vi "Drfit_check.vi"() -> ()   [LabVIEW 2019]
uses:
  <vilib>/eio/EIONode/EIONode.xnode
  <vilib>/rvi/eio/common/nirviEmuTemplateMethod_errors.vi
  <vilib>/rvi/DataTransferAndStorage/Container/XNode/niFpgaContainer.xnode
  <vilib>/rvi/FIFO/Fifo_Resource/nirvififoEmulationRead.vi
  <vilib>/eio/EIOPropertyNode/EIOPropertyNode.xnode
  <vilib>/rvi/eio/common/nirviEmuTemplatePropertyGet_errors.vi
  <vilib>/rvi/eio/common/nirviEmuTemplatePropertyGet_noerrors.vi
  <vilib>/rvi/eio/common/nirviEmuTemplatePropertySet_errors.vi
  <vilib>/rvi/eio/common/nirviEmuTemplatePropertySet_noerrors.vi
  <vilib>/rvi/FIFO/Fifo_Resource/nirvififoEmulationWrite.vi
  <vilib>/rvi/interface/RandomDataEmulation/nirviRandomDataFpgaReadWriteTemplate.vi
panel:
  in  "MobX(px/V)":sgl
  in  "1/Xcali":sgl
  in  "Xmean":sgl
  in  "Frequency":u32=100000
  in  "Triangle wave":T1={"signal offset_X"=5.0, "Scale X"=0.0, "signal offset_Y"=5.0, "Scale Y"=0.0, "Phase Shift"=30}
  in  "1/Ycali":sgl
  in  "Xoffset":sgl
  in  "Yoffset":sgl
  in  "sum_offset":sgl
  in  "Normalize signal":bool=TRUE
  in  "FB Time":u8=5 caption="Feedback loop time"
  out "Saveloop":u32
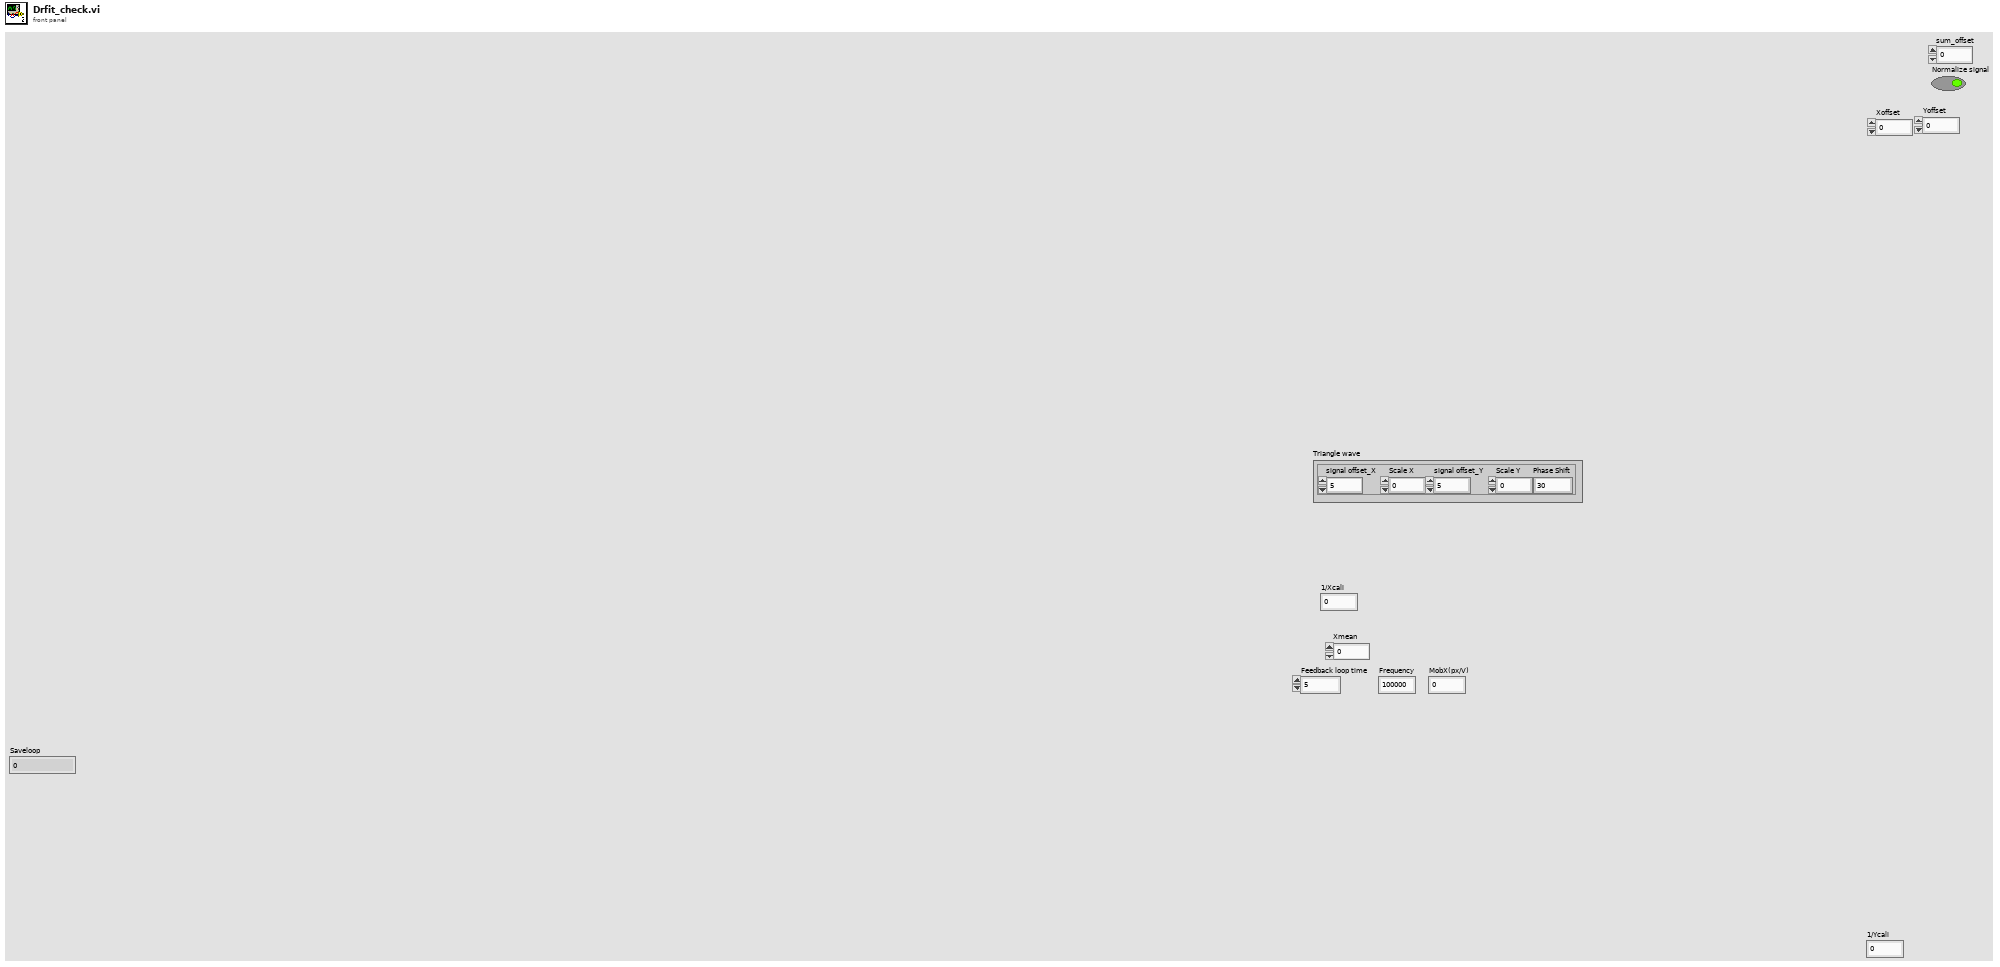
[diagram p1: front panel]
types:
  T1 = cluster{"signal offset_X":sgl, "Scale X":sgl, "signal offset_Y":sgl, "Scale Y":sgl, "Phase Shift":u32}
  T2 = enum8{"+/- 10 V", "+/- 5 V", "+/- 2 V", "+/- 1 V"}
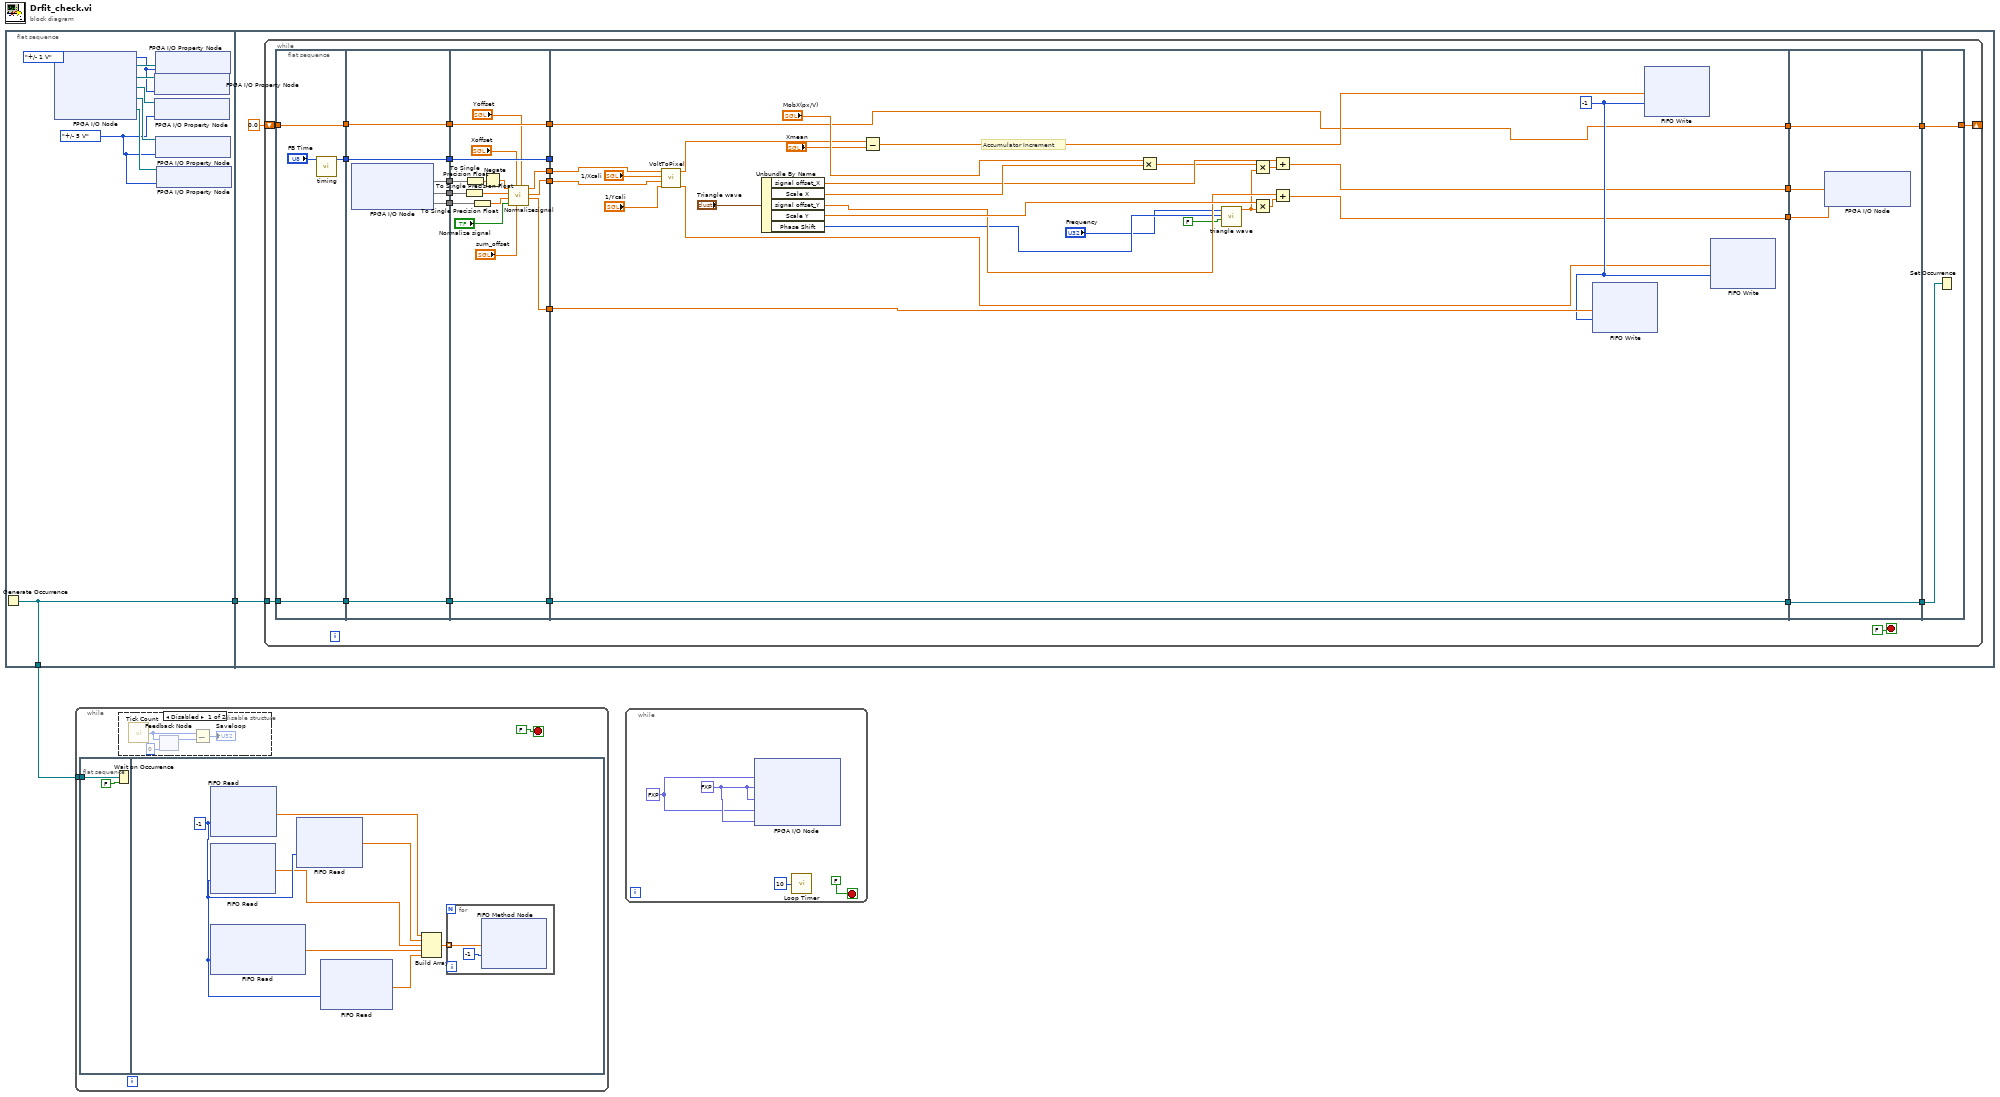
[diagram p0: block diagram]
diagram:
  n1 = flat-sequence {
    tunnel: [w3] -> w2
    tunnel: [w3] -> w1
    tunnel: w2 -> [w12]
    frame #0 {
      w4 = T2."+/- 5 V" ("Voltage Range")
      w7 = T2."+/- 1 V" ("Voltage Range")
      n2 = Generate Occurrence() -> (w3:refnum<k4>)
      n3 = xnode "FPGA I/O Node"() -> ("FPGA I/O Out"=w10:refnum<k21>, "FPGA I/O Out"=w8:refnum<k21>, "FPGA I/O Out"=w9:refnum<k21>, "FPGA I/O Out"=w5:refnum<k21>, "FPGA I/O Out"=w6:refnum<k21>)  [unwired: 5 in, 5 out]
      n4 = xnode "FPGA I/O Property Node"("FPGA I/O In"=w8, "Voltage Range"=w7) -> ()  [unwired: 1 out]
      n5 = xnode "FPGA I/O Property Node"("FPGA I/O In"=w9, "Voltage Range"=w4) -> ()  [unwired: 1 out]
      n6 = xnode "FPGA I/O Property Node"("FPGA I/O In"=w10, "Voltage Range"=w7) -> ()  [unwired: 1 out]
      n7 = xnode "FPGA I/O Property Node"("FPGA I/O In"=w5, "Voltage Range"=w4) -> ()  [unwired: 1 out]
      n8 = xnode "FPGA I/O Property Node"("FPGA I/O In"=w6, "Voltage Range"=w4) -> ()  [unwired: 1 out]
    }
    frame #1 {
      n9 = while {
        tunnel: w12 -> [w25]
        shift-right: [w17] -> _
        shift-left: sgl 0.0 -> [w15]
        stop <- FALSE ("stop") stop-if-true
        n10 = flat-sequence {
          tunnel: [w40] -> w26
          tunnel: w25 -> [w39]
          tunnel: [w39] -> w24
          tunnel: [w38] -> w16
          tunnel: w15 -> [w38]
          tunnel: [w47] -> w36
          tunnel: [w46] -> w34
          tunnel: [w45] -> w32
          tunnel: [w44] -> w27
          tunnel: w26 -> [w44]
          tunnel: w24 -> [w43]
          tunnel: [w43] -> w23
          tunnel: w16 -> [w42]
          tunnel: [w42] -> w13
          tunnel: w36 -> [w54]
          tunnel: [w63] -> w35
          tunnel: w34 -> [w53]
          tunnel: [w62] -> w33
          tunnel: w32 -> [w51]
          tunnel: [w61] -> w31
          tunnel: [w64] -> w28
          tunnel: w27 -> [w64]
          tunnel: w23 -> [w60]
          tunnel: [w60] -> w22
          tunnel: [w58] -> w14
          tunnel: w13 -> [w58]
          tunnel: w35 -> [w90]
          tunnel: w33 -> [w73]
          tunnel: w31 -> [w89]
          tunnel: [w74] -> w30
          tunnel: [w71] -> w29
          tunnel: w28 -> [_]
          tunnel: w22 -> [w87]
          tunnel: [w87] -> w20
          tunnel: [w82] -> w19
          tunnel: w14 -> [w82]
          tunnel: w29 -> [w94]
          tunnel: w30 -> [w95]
          tunnel: [w93] -> w21
          tunnel: w20 -> [w93]
          tunnel: w19 -> [w92]
          tunnel: [w92] -> w18
          tunnel: w21 -> [w97]
          tunnel: [w96] -> w17
          tunnel: w18 -> [w96]
          frame #0 {
            n11 = call "timing.vi"("Feedback loop time"="FB Time") -> ("Feedback Loop time"=w40:u32)  [unwired: 10 in]
          }
          frame #1 {
            n12 = xnode "FPGA I/O Node"() -> ("Connector1/AI2"=w47, "Connector1/AI4"=w46, "Connector1/AI5"=w45)  [unwired: 3 in, 3 out]
          }
          frame #2 {
            n13 = To Single Precision Float(number=w53) -> (single precision float=w52:sgl)
            n14 = To Single Precision Float(number=w54) -> (single precision float=w49:sgl)
            n15 = To Single Precision Float(number=w51) -> (single precision float=w50:sgl)
            n16 = Negate(x=w49) -> (-x=w48:sgl)
            n17 = call "Normalizesignal.vi"("Yoffset"="Yoffset", "sum_offset"="sum_offset", "Xoffset"="Xoffset", "Normalize signal"="Normalize signal", "Sum"=w50, "Y"=w52, "X"=w48) -> ("Sum"=w61:sgl, "Y"=w62:sgl, "X"=w63:sgl)  [unwired: 2 in]
          }
          frame #3 {
            w83 = -1 ("Timeout")
            # "Accumulator Increment"
            n18 = call "VoltToPixel.vi"("1/(QPDY/px)"="1/Ycali", "Normalized Y"=w73, "1/(QPDX/px)"="1/Xcali", "Normalized X"=w90) -> ("Ypx"=w75:sgl, "Xpx"=w86:sgl)  [unwired: 6 in]
            n19 = Unbundle By Name("Triangle wave") -> ("signal offset_X"=w78:sgl, "Scale X"=w80:sgl, "signal offset_Y"=w77:sgl, "Scale Y"=w79:sgl, "Phase Shift"=w76:u32)
            n20 = Subtract(x=w86, y="Xmean") -> (x-y=w88:sgl)
            n21 = Multiply(x="MobX(px/V)", y=w80) -> (x*y=w69:sgl)
            n22 = call "triangle wave.vi"("Reset Accumulator_TW"=FALSE, "phase shift"=w76, "Frequency"="Frequency") -> ("Tri wave out"=w66:sgl)  [unwired: 8 in]
            n23 = Multiply(x=w69, y=w66) -> (x*y=w68:sgl)
            n24 = Multiply(x=w79, y=w66) -> (x*y=w70:sgl)
            n25 = Add(x=w78, y=w68) -> (x+y=w74:sgl)
            n26 = Add(x=w77, y=w70) -> (x+y=w71:sgl)
            n27 = xnode ("FIFO Write")("Element"=w89, "Timeout"=w83) -> ()  [unwired: 1 in, 2 out]
            n28 = xnode ("FIFO Write")("Element"=w88, "Timeout"=w83) -> ()  [unwired: 1 in, 2 out]
            n29 = xnode ("FIFO Write")("Element"=w75, "Timeout"=w83) -> ()  [unwired: 1 in, 2 out]
          }
          frame #4 {
            n30 = xnode "FPGA I/O Node"("Connector1/AO7"=w95, "Connector1/AO6"=w94) -> ()  [unwired: 2 in, 2 out]
          }
          frame #5 {
            n31 = Set Occurrence(w97) -> ()
          }
        }
      }
    }
  }
  n32 = while {
    tunnel: w1 -> [w98]
    stop <- FALSE stop-if-true
    n33 = flat-sequence {
      tunnel: w98 -> [w105]
      frame #0 {
        n34 = Wait on Occurrence(1:FALSE ("ignore previous (T)"), 2:w105) -> ()  [unwired: 1 in, 1 out]
      }
      frame #1 {
        w108 = -1 ("Timeout")
        n35 = xnode ("FIFO Read")("Timeout"=w108) -> ("Element"=w106:sgl)  [unwired: 1 in, 2 out]
        n36 = xnode ("FIFO Read")("Timeout"=w108) -> ("Element"=w109:sgl)  [unwired: 1 in, 2 out]
        n37 = xnode ("FIFO Read")("Timeout"=w108) -> ("Element"=w110:sgl)  [unwired: 1 in, 2 out]
        n38 = xnode ("FIFO Read")("Timeout"=w108) -> ("Element"=w107:sgl)  [unwired: 1 in, 2 out]
        n39 = xnode ("FIFO Read")("Timeout"=w108) -> ("Element"=w111:sgl)  [unwired: 1 in, 2 out]
        n40 = Build Array(w110, w107, w106, w109, w111) -> (w112:sgl[])
        n41 = for {
          tunnel: w112 -> [w114] mode=indexing
          n42 = xnode ("FIFO Method Node")("Element"=w114, "Timeout"=-1) -> ()  [unwired: 1 in, 2 out]
        }
      }
    }
    n43 = disable-structure shown="Disabled" {
      frame Disabled {
        n44 = call "Tick Count"() -> ("Tick Count(uSec)"=w103:u32)
        n45 = feedback #1(u32 0 ("Tick Count(uSec)")) -> (w102:u32)
        n46 = feedback-in #1(w103) -> ()
        n47 = Subtract(x=w103, y=w102) -> (x-y=→"Saveloop":u32)
      }
      frame Enabled {
      }
    }
  }
  n48 = while {
    stop <- FALSE stop-if-true
    w115 = fxp<+,8,3> 2.5 ("Connector1/AO2")
    w116 = fxp<+,8,3> 5.0 ("Connector1/AO2")
    n49 = xnode "FPGA I/O Node"("Connector1/AO0"=w115, "Connector1/AO2"=w116, "Connector1/AO3"=w116, "Connector1/AO4"=w115, "Connector1/AO5"=w116) -> ()  [unwired: 5 in, 5 out]
    n50 = call "Loop Timer"("Count(uSec)"=u8 10) -> ()  [unwired: 1 out]
  }
